vi "New Protected Subpanel.vi"(10 "Panel Transparent? (T)":bool=TRUE, 11 "SubPnl Refnum":refnum<vi>) -> (0 "error out":errorcluster, 3 "Protected Subpanel":T1)   [LabVIEW 2020, in "IViewable.lvlib" / "ProtectedSubpanel.lvclass"]
doc: "新建受保护子面板"
uses:
  ProtectedSubpanel.lvclass
  Protected Subpanel Reference.ctl
  ProtectedSubpanel.lvclass/ProtectedSubpanel.ctl
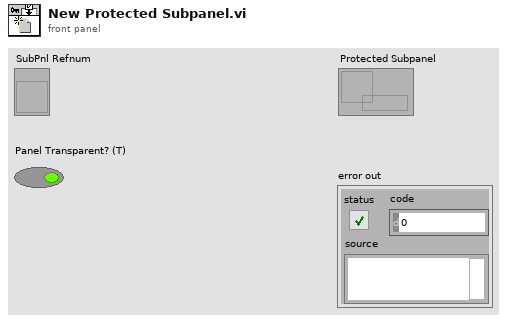
[diagram p1: front panel]
types:
  T1 = typedef "IViewable.lvlib/ProtectedSubpanel.lvclass/Protected Subpanel Reference.ctl" = refnum<data-value>
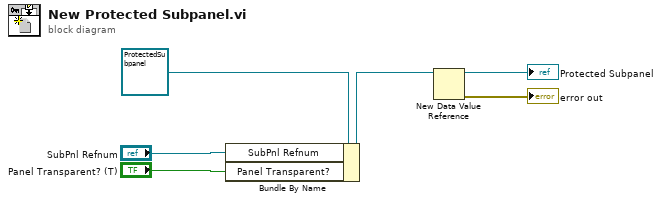
[diagram p0: block diagram]
diagram:
  n1 = Bundle By Name(cluster=refnum<class "ProtectedSubpanel.lvclass"> refnum ("ProtectedSubpanel in"), "SubPnl Refnum"="SubPnl Refnum", "Panel Transparent?"="Panel Transparent? (T)") -> (w4:refnum<class "ProtectedSubpanel.lvclass">)
  n2 = New Data Value Reference(data value=w4) -> (data value reference=→"Protected Subpanel":refnum<data-value>, error out=→"error out":errorcluster)  [unwired: 1 in]
